vi "StartCircBufferAcq.vi"(8 "error in (no error)":errorcluster, 10 "exp_time":u32=100, 11 "hCam":i16) -> (0 "error out":errorcluster, 2 "stream_size":u32, 3 "image buff":u16[](array[numeric]))   [LabVIEW 2021]
uses:
  Low_level_subVIs/PVCAM_rgn_type.ctl
panel:
  out "return type":i16
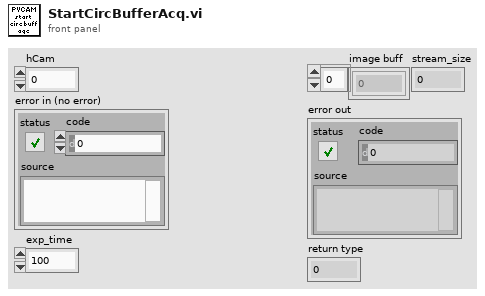
[diagram p1: front panel]
types:
  T1 = enum16{"ATTR_CURRENT", "ATTR_COUNT", "ATTR_TYPE", "ATTR_MIN", "ATTR_MAX", "ATTR_DEFAULT", "ATTR_INCREMENT", "ATTR_ACCESS", "ATTR_AVAIL"}
  T2 = enum16{"CIRC_NONE", "CIRC_OVERWRITE", "CIRC_NO_OVERWRITE"}
  T3 = typedef "PVCAM_rgn_type.ctl" = cluster{"s1":u16, "s2":u16, "sbin":u16, "p1":u16, "p2":u16, "pbin":u16}
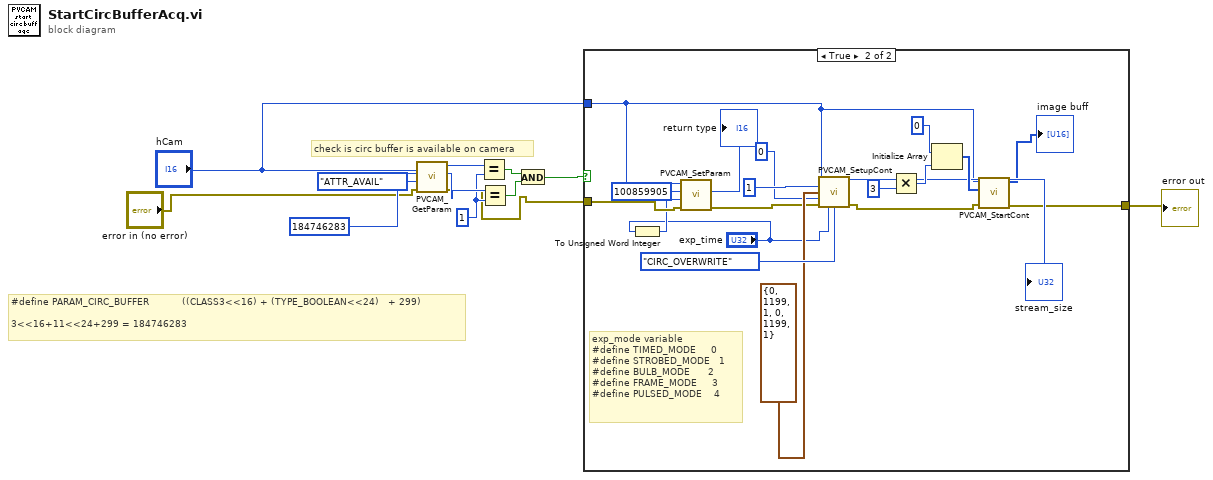
[diagram p0: block diagram]
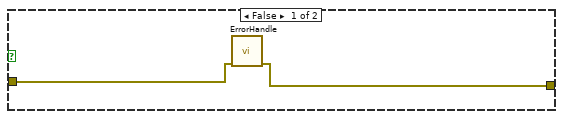
[diagram p2: hidden frame]
diagram:
  w8 = i16 1 ("y")
  # "check is circ buffer is available on camera"
  # "#define PARAM_CIRC_BUFFER           ((CLASS3<<16) + (TYPE_BOOLEAN<<24)   + 299)\n\n3<<16+11<<24+299 = 184746283"
  n1 = call "PVCAM_GetParam.vi"("error in (no error)"="error in (no error)", "param_attrib"=T1."ATTR_AVAIL", "param_id"=u32 184746283, "hCam"="hCam") -> ("error out"=w4:errorcluster, "return type"=w9:i16, "param_value"=w11:i16)  [unwired: 5 in]
  n2 = Equal?(x=w11, y=w8) -> (x = y?=w10:bool)
  n3 = Equal?(x=w9, y=w8) -> (x = y?=w7:bool)
  n4 = And(x=w10, y=w7) -> (x .and. y?=w3:bool)
  n5 = case shown="True" w3 {
    tunnel: w4 -> [w14 w21]
    tunnel: "hCam" -> [_ w19]
    tunnel: [w13 w22] -> w1
    frame False {
      n6 = call "ErrorHandle.vi"("error in (no error)"=w14) -> ("error in (no error) 2"=w13:errorcluster)  [unwired: 10 in]
    }
    frame True {
      # "exp_mode variable\n#define TIMED_MODE     0\n#define STROBED_MODE   1\n#define BULB_MODE      2\n#define FRAME_MODE     3\n#define PULSED_MODE    4"
      n7 = To Unsigned Word Integer(number="exp_time") -> (unsigned 16bit integer=w18:u16)
      n8 = call "PVCAM_SetParam.vi"("error in (no error)"=w21, "param_value"=w18, "param_id"=u32 100859905, "hCam"=w19) -> ("error out"=w20:errorcluster, "return type"=→"return type":i16)  [unwired: 6 in]
      n9 = call "PVCAM_SetupCont.vi"("hCam"=w19, "rgn_total"=u16 1 ("exp_total"), "rgn_type"=T3 {"s1"=0, "s2"=1199, "sbin"=1, "p1"=0, "p2"=1199, "pbin"=1}, "exp_mode"=i16 0, "error in (no error)"=w20, "exp_time"="exp_time", "circ_mode"=T2."CIRC_OVERWRITE") -> ("stream_size"=w25:u32, "error out"=w27:errorcluster)  [unwired: 6 in, 1 out]
      "stream_size" <- w25
      n10 = Multiply(x=w25, y=u32 3) -> (x*y=w29:u32)
      n11 = Initialize Array(u16 0 ("element"), w29) -> (w28:u16[])
      n12 = call "PVCAM_StartCont.vi"("error in (no error)"=w27, "buffer"=w28, "hCam"=w19) -> ("error out"=w22:errorcluster, "ImageBuf"=→"image buff":u8[])  [unwired: 6 in, 1 out]
    }
  }
  "error out" <- w1
